vi "Build Update.vi"(8 "error in (no error)":errorcluster, 9 "tableName":string, 10 "DynamicParameters in":refnum<class "DynamicParameters.lvclass">, 11 "DbConnection in":refnum<class "DbConnection.lvclass">) -> (0 "error out":errorcluster, 2 "Query":string, 3 "DbConnection out":refnum<class "DbConnection.lvclass">)   [LabVIEW 2020, in "ORM.lvlib" / "DbConnection.lvclass"]
uses:
  DbConnection.lvclass
  DynamicParameters/DynamicParameters.lvclass
  DbConnection.lvclass/DbConnection.ctl
  DynamicParameters/DynamicParameters.lvclass/DynamicParameters.ctl
  Read ColumnNameEqualsValueFormat.vi
  DynamicParameters/Read FieldNames.vi
  DynamicParameters/Read ParameterNames.vi
  DynamicParameters/Read KeyProperties.vi
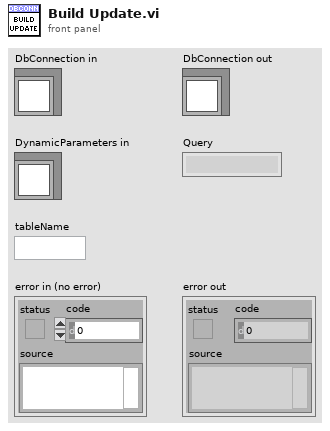
[diagram p1: front panel]
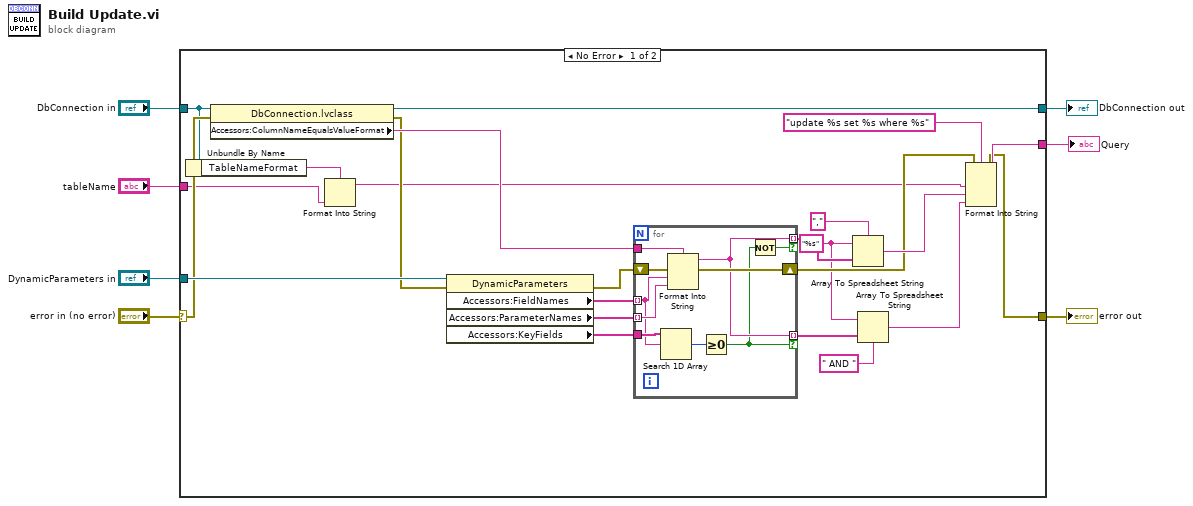
[diagram p0: block diagram]
diagram:
  n1 = case shown="No Error" "error in (no error)" {
    selector: "error in (no error)" -> [w22 w43]
    tunnel: [w18 w43] -> w6
    tunnel: [w31 w42] -> w4
    tunnel: "DbConnection in" -> [w11 w42]
    tunnel: "DynamicParameters in" -> [w30 _]
    tunnel: "tableName" -> [w9 _]
    tunnel: [w23 _] -> w1
    frame No Error {
      w15 = "%s" ("format string")
      n2 = Unbundle By Name(w11) -> ("TableNameFormat"=w10:string)
      n3 = property class="DbConnection.lvclass"(reference=w11, error in=w22) -> (reference out=w31:refnum<class "DbConnection.lvclass">, error out=w21:errorcluster, "Accessors:ColumnNameEqualsValueFormat"=w27:string)
      n4 = Format Into String(format string=w10, w9) -> (resulting string=w8:string)  [unwired: 2 in, 1 out]
      n5 = property class="DynamicParameters"(reference=w30, error in=w21) -> (error out=w20:errorcluster, "Accessors:FieldNames"=w29:string[], "Accessors:ParameterNames"=w28:string[], "Accessors:KeyFields"=w17:string[])  [unwired: 1 out]
      n6 = for {
        tunnel: w29 -> [w36] mode=indexing
        tunnel: w28 -> [w40] mode=indexing
        tunnel: w27 -> [w41]
        tunnel: [w34] -> w24 mode=indexing if=w32
        shift-right: [w38] -> w19
        shift-left: w20 -> [w39]
        tunnel: w17 -> [w37]
        tunnel: [w34] -> w16 mode=indexing if=w33
        n7 = Search 1D Array(1D array=w37, element=w36) -> (index of element=w35:i32)  [unwired: 1 in]
        n8 = Format Into String(format string=w41, error in=w39, w36, w40) -> (resulting string=w34:string, error out=w38:errorcluster)  [unwired: 1 in]
        n9 = Greater Or Equal To 0?(x=w35) -> (x >= 0?=w33:bool)
        n10 = Not(x=w33) -> (.not. x?=w32:bool)
      }
      n11 = Array To Spreadsheet String(delimiter (Tab)=",", array=w24, 3:w15) -> (spreadsheet string=w25:string)
      n12 = Array To Spreadsheet String(delimiter (Tab)=" AND ", array=w16, 3:w15) -> (spreadsheet string=w13:string)
      n13 = Format Into String(format string="update %s set %s where %s", error in=w19, w8, w25, w13) -> (resulting string=w23:string, error out=w18:errorcluster)  [unwired: 1 in]
    }
    frame Error {
    }
  }
  "error out" <- w6
  "DbConnection out" <- w4
  "Query" <- w1
